vi "S2C_PCIe7841_Poly_HandSwitchRead.vi"(8 "Error In":errorcluster, 10 "HandSwitch":cluster{"HandSwitch":T1}={"HandSwitch"="220"}, 11 "Settings":T2={"Driver"="PCIe7841", "Command"="HandSwitchRead", "Return"="State", "Parameters"="", "Timeout"=10.0}) -> (0 "Error Out":errorcluster, 3 "Response":string)   [LabVIEW 2015]
uses:
  Typedefs/S2C_PCIe7841_Type_HandSwitchRd.ctl
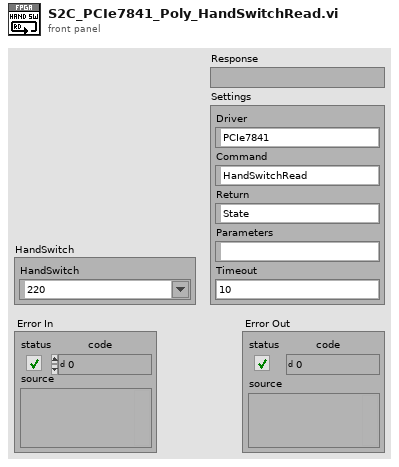
[diagram p1: front panel]
types:
  T1 = typedef "S2C_PCIe7841_Type_HandSwitchRd.ctl" = string
  T2 = cluster{"Driver":string, "Command":string, "Return":string, "Parameters":string, "Timeout":dbl}
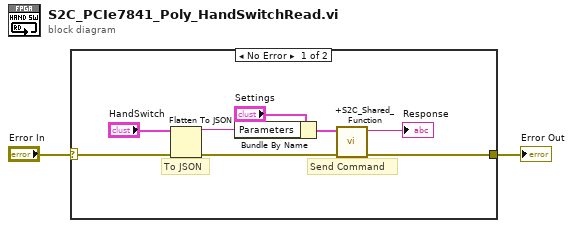
[diagram p0: block diagram]
diagram:
  n1 = case shown="No Error" "Error In" {
    selector: "Error In" -> [w6 w11]
    tunnel: [w5 w11] -> w1
    frame No Error {
      # "To JSON"
      # "Send Command"
      n2 = Flatten To JSON(anything="HandSwitch", error in (no error)=w6) -> (JSON string=w7:string, 11:w9:errorcluster)  [unwired: 1 in]
      n3 = Bundle By Name(cluster="Settings", "Parameters"=w7) -> (w10:T2)
      n4 = call "+S2C_Shared_Function.vi"("Error In"=w9, "Settings"=w10) -> ("Error Out"=w5:errorcluster, "Response"=→"Response":string)  [unwired: 8 in]
    }
    frame Error {
    }
  }
  "Error Out" <- w1
